vi "monitor registers.vi"(7 "register monitor queue":refnum<queue>, 8 "error in":errorcluster, 9 "Registers":T1[](array[typedef]), 10 "bus instance name":string, 11 "fpga interface in":refnum<k20>) -> (0 "error out":errorcluster, 3 "fpga interface out":refnum<k20>, 5 "register monitor queue out":refnum<queue>)   [LabVIEW 2025, in "Automotive Vision.lvclass"]
uses:
  Automotive Vision.lvclass
  Automotive Vision.lvclass/Automotive Vision.ctl
  <instrlib>/FlexRIO/API/Host/v1/NI FlexRIO API v1.lvlib
  regitster_value.ctl
  register.ctl
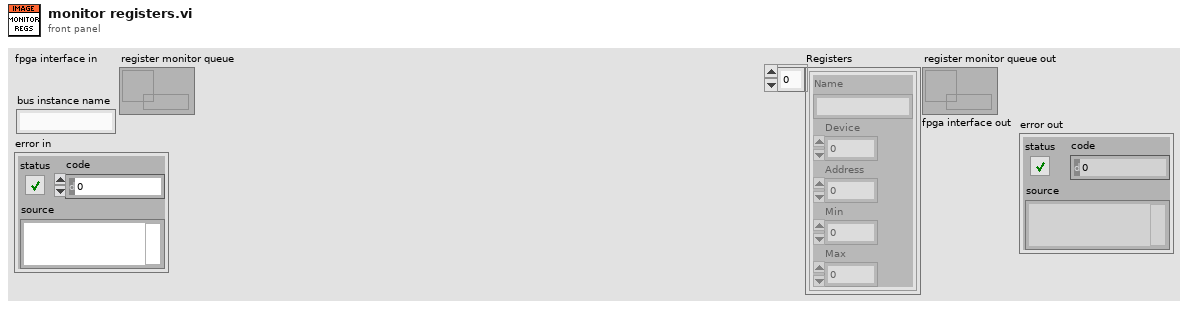
[diagram p1: front panel]
types:
  T1 = typedef "Automotive Vision.lvclass/register.ctl" = cluster{"Name":string, "Device":u8, "Address":u16, "Min":u16, "Max":u16}
  T2 = typedef "Automotive Vision.lvclass/regitster_value.ctl" = cluster{"Source":u8, "Address":u16, "Value":u16}
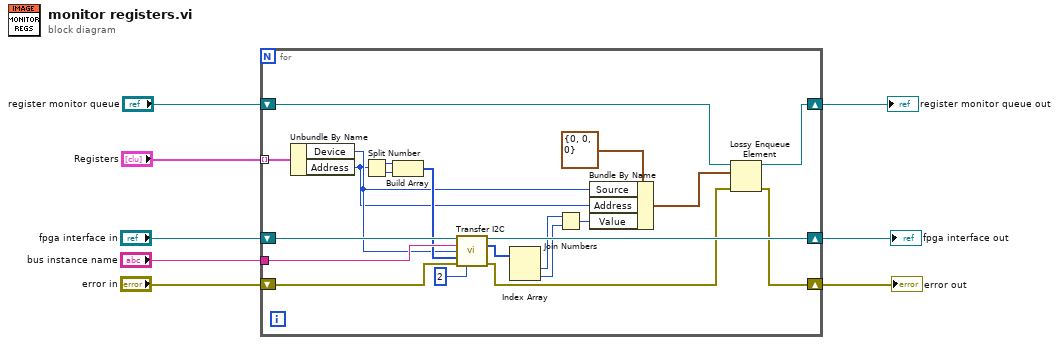
[diagram p0: block diagram]
diagram:
  n1 = for {
    tunnel: "Registers" -> [w29] mode=indexing
    tunnel: "bus instance name" -> [w27]
    shift-right: [w9] -> w1
    shift-left: "error in" -> [w23]
    shift-right: [w21] -> w2
    shift-left: "fpga interface in" -> [w28]
    shift-right: [w11] -> w3
    shift-left: "register monitor queue" -> [w13]
    n2 = Unbundle By Name(w29) -> ("Device"=w19:u8, "Address"=w18:u16)
    n3 = Split Number(x=w18) -> (hi(x)=w26:u8, lo(x)=w25:u8)
    n4 = Build Array(w26, w25) -> (w24:u8[])
    n5 = call <instrlib>:"Transfer I2C.vi"("fpga interface in"=w28, "bus instance name"=w27, "slave address"=w19, "write data"=w24, "error in"=w23, "num bytes to read"=u32 2) -> ("fpga interface out"=w21:refnum<k20>, "read data"=w16:u8[], "error out"=w10:errorcluster)  [unwired: 6 in, 1 out]
    n6 = Index Array(array=w16) -> (element #1=w15:u8, element #2=w14:u8)  [unwired: 2 in]
    n7 = Join Numbers(hi=w15, lo=w14) -> ((hi.lo)=w17:u16)
    n8 = Bundle By Name(cluster=T2 {"Source"=0, "Address"=0, "Value"=0} ("Register Value"), "Source"=w19, "Address"=w18, "Value"=w17) -> (w12:T2)
    n9 = Lossy Enqueue Element(queue=w13, element=w12, error in (no error)=w10) -> (queue out=w11:refnum<queue>, error out=w9:errorcluster)  [unwired: 2 out]
  }
  "register monitor queue out" <- w3
  "fpga interface out" <- w2
  "error out" <- w1
